vi "XML readSamplesFromXML.getTXAttributes.vi"(9 "TXSelect (TX1":enum16{"TX1", "TX2"}(ring), 10 "Sample XML":string, 11 "Sample in":T1) -> (3 "Sample out":T1)   [LabVIEW 2011]
uses:
  Controls/PIM.API.Response.Samples.ctl
  iQA Sweep Behavior.ctl
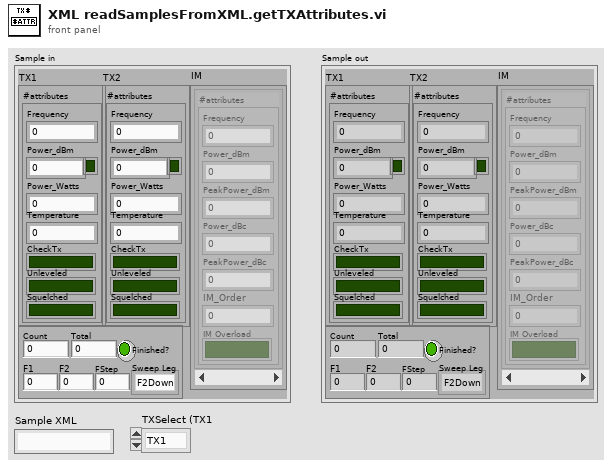
[diagram p1: front panel]
types:
  T1 = typedef "PIM.API.Response.Samples.ctl" = cluster{"TX1":cluster{"#attributes":cluster{"Frequency":dbl, "Power_dBm":dbl, "Power_Watts":dbl, "CheckTx":bool, "Unleveled":bool, "Squelched":bool, "Temperature":dbl, "ToneOn":bool}}, "TX2":cluster{"#attributes":cluster{"Frequency":dbl, "Power_dBm":dbl, "Power_Watts":dbl, "CheckTx":bool, "Unleveled":bool, "Squelched":bool, "Temperature":dbl, "ToneOn":bool}}, "IM":cluster{"#attributes":cluster{"Frequency":dbl, "Power_dBm":dbl, "PeakPower_dBm":dbl, "Power_dBc":dbl, "PeakPower_dBc":dbl, "IM_Order":u8, "IM Overload":bool}}[], "#attributes":cluster{"Count":u32, "Total":u32, "Finished?":bool, "Sweep Leg":T2, "F1":dbl, "F2":dbl, "FStep":dbl}}
  T2 = typedef "iQA Sweep Behavior.ctl" = enum16{"F2Down", "F1Up", "RxMultiIM"}
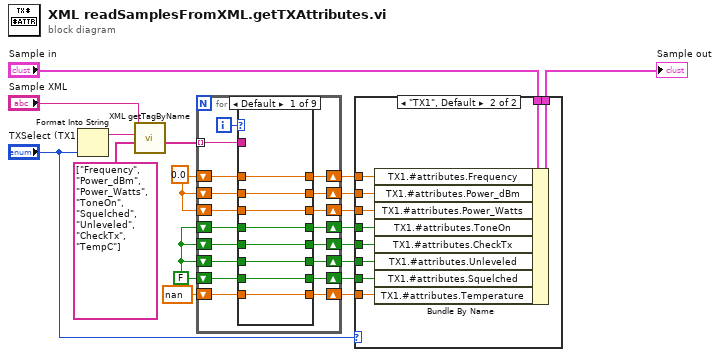
[diagram p0: block diagram]
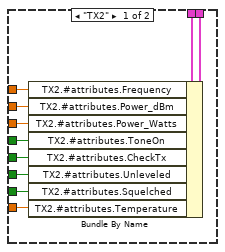
[diagram p2: hidden frame]
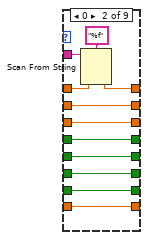
[diagram p3: hidden frame]
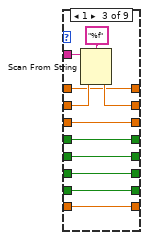
[diagram p4: hidden frame]
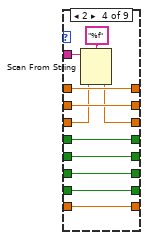
[diagram p5: hidden frame]
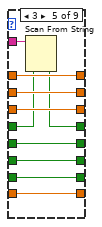
[diagram p6: hidden frame]
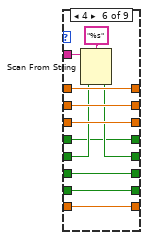
[diagram p7: hidden frame]
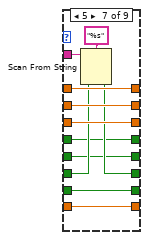
[diagram p8: hidden frame]
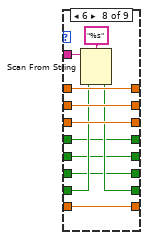
[diagram p9: hidden frame]
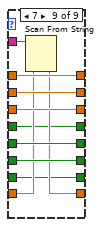
[diagram p10: hidden frame]
diagram:
  w1 = FALSE
  w6 = 0.0
  n1 = Format Into String("TXSelect (TX1") -> (resulting string=w16:string)  [unwired: 3 in, 1 out]
  n2 = call "XML getTagByName.vi"("Get Attributes"=string[] ["Frequency", "Power_dBm", "Power_Watts", "ToneOn", "Squelched", "Unleveled", "CheckTx", "TempC"], "Tag Name"=w16, "XML String"="Sample XML") -> ("Attribute Values"=w18:string[])  [unwired: 4 in, 4 out]
  n3 = for {
    shift-right: [w35] -> w14
    shift-left: w6 -> [w32]
    shift-right: [w34] -> w13
    shift-left: w6 -> [w33]
    shift-right: [w30] -> w12
    shift-left: w6 -> [w31]
    tunnel: w18 -> [w29] mode=indexing
    shift-right: [w25] -> w11
    shift-left: w1 -> [w28]
    shift-right: [w24] -> w10
    shift-left: w1 -> [w27]
    shift-right: [w23] -> w9
    shift-left: w1 -> [w26]
    shift-right: [w21] -> w3
    shift-left: nan -> [w22]
    shift-right: [w20] -> w2
    shift-left: w1 -> [w19]
    i -> [w36]
    n4 = case shown="Default" w36 {
      tunnel: [w44 w54 w62 w75 w86 w96 w107 w118 w129] -> w35
      tunnel: [w43 w52 w65 w76 w87 w97 w108 w119 w130] -> w34
      tunnel: w33 -> [w43 w52 w64 w76 w87 w97 w108 w119 w130]
      tunnel: w32 -> [w44 w53 w62 w75 w86 w96 w107 w118 w129]
      tunnel: w31 -> [w42 w51 w63 w74 w80 w94 w105 w116 w127]
      tunnel: [w42 w51 w63 w73 w80 w94 w105 w116 w127] -> w30
      tunnel: w29 -> [_ w50 w61 w72 w85 w95 w106 w117 w128]
      tunnel: w28 -> [w41 w49 w60 w71 w84 w93 w102 w113 w126]
      tunnel: w27 -> [w40 w48 w59 w70 w83 w91 w104 w112 w125]
      tunnel: w26 -> [w39 w47 w58 w69 w82 w90 w101 w115 w122]
      tunnel: [w41 w49 w60 w71 w84 w92 w102 w113 w126] -> w25
      tunnel: [w40 w48 w59 w70 w83 w91 w103 w112 w125] -> w24
      tunnel: [w39 w47 w58 w69 w82 w90 w101 w114 w122] -> w23
      tunnel: w22 -> [w38 w46 w57 w68 w81 w89 w100 w111 w124]
      tunnel: [w38 w46 w57 w68 w81 w89 w100 w111 w123] -> w21
      tunnel: w19 -> [w37 w45 w56 w67 w79 w88 w99 w110 w121]
      tunnel: [w37 w45 w56 w67 w78 w88 w99 w110 w121] -> w20
      frame Default {
      }
      frame 0 {
        n5 = Scan From String(format string="%f", input string=w50, default 1=w53) -> (output 1=w54:dbl)  [unwired: 2 in, 3 out]
      }
      frame 1 {
        n6 = Scan From String(format string="%f", input string=w61, default 1=w64) -> (output 1=w65:dbl)  [unwired: 2 in, 3 out]
      }
      frame 2 {
        n7 = Scan From String(format string="%f", input string=w72, default 1=w74) -> (output 1=w73:dbl)  [unwired: 2 in, 3 out]
      }
      frame 3 {
        n8 = Scan From String(input string=w85, default 1=w79) -> (output 1=w78:bool)  [unwired: 3 in, 3 out]
      }
      frame 4 {
        n9 = Scan From String(format string="%s", input string=w95, default 1=w93) -> (output 1=w92:bool)  [unwired: 2 in, 3 out]
      }
      frame 5 {
        n10 = Scan From String(format string="%s", input string=w106, default 1=w104) -> (output 1=w103:bool)  [unwired: 2 in, 3 out]
      }
      frame 6 {
        n11 = Scan From String(format string="%s", input string=w117, default 1=w115) -> (output 1=w114:bool)  [unwired: 2 in, 3 out]
      }
      frame 7 {
        n12 = Scan From String(input string=w128, default 1=w124) -> (output 1=w123:dbl)  [unwired: 3 in, 3 out]
      }
    }
  }
  n13 = case shown="\"TX1\", Default" "TXSelect (TX1" {
    tunnel: w14 -> [w140 w150]
    tunnel: w13 -> [w139 w149]
    tunnel: w12 -> [w138 w148]
    tunnel: w11 -> [w137 w147]
    tunnel: w10 -> [w136 w146]
    tunnel: w9 -> [w135 w145]
    tunnel: [w133 w144] -> w8
    tunnel: "Sample in" -> [w134 w143]
    tunnel: w3 -> [w132 w142]
    tunnel: w2 -> [w131 w141]
    frame "TX2" {
      n14 = Bundle By Name(cluster=w134, "TX2.#attributes.Frequency"=w140, "TX2.#attributes.Power_dBm"=w139, "TX2.#attributes.Power_Watts"=w138, "TX2.#attributes.ToneOn"=w131, "TX2.#attributes.CheckTx"=w137, "TX2.#attributes.Unleveled"=w136, "TX2.#attributes.Squelched"=w135, "TX2.#attributes.Temperature"=w132) -> (w133:T1)
    }
    frame "TX1", Default {
      n15 = Bundle By Name(cluster=w143, "TX1.#attributes.Frequency"=w150, "TX1.#attributes.Power_dBm"=w149, "TX1.#attributes.Power_Watts"=w148, "TX1.#attributes.ToneOn"=w141, "TX1.#attributes.CheckTx"=w147, "TX1.#attributes.Unleveled"=w146, "TX1.#attributes.Squelched"=w145, "TX1.#attributes.Temperature"=w142) -> (w144:T1)
    }
  }
  "Sample out" <- w8
